vi "onenote_dialogue.vi"(8 "error in (no error)":errorcluster, 11 "Image Path":path=path "C:/Users/monke/Desktop/Work/VIs to modify/ONENOTE/Sandbox/TEST.BMP") -> (0 "error out":errorcluster, 2 "Description Out":string, 3 "Image Path Out":path)   [LabVIEW 2016]
uses:
  <vilib>/Utility/miscctls.llb/LVBoundsTypeDef.ctl
panel:
  in  "Options_Cluster":T1
  in  "Options":bool
  out "new picture":picture
  in  "Description":string="Write your description here. \nTo make text bold in OneNote, surround with <b><b/> tags.\nTo make text bold in OneNote, surround with <i><i/> tags."
  in  "Finish":bool
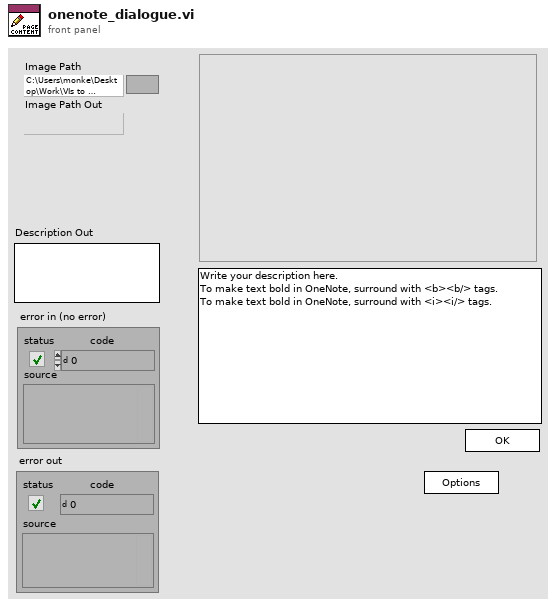
[diagram p1: front panel]
types:
  T1 = cluster{"Strikethrough":bool, "SubScript":bool, "Italics":bool, "Bold":bool, "SuperScript":bool}
  T2 = typedef "LVBoundsTypeDef.ctl" = cluster{"Width":u32, "Height":u32}
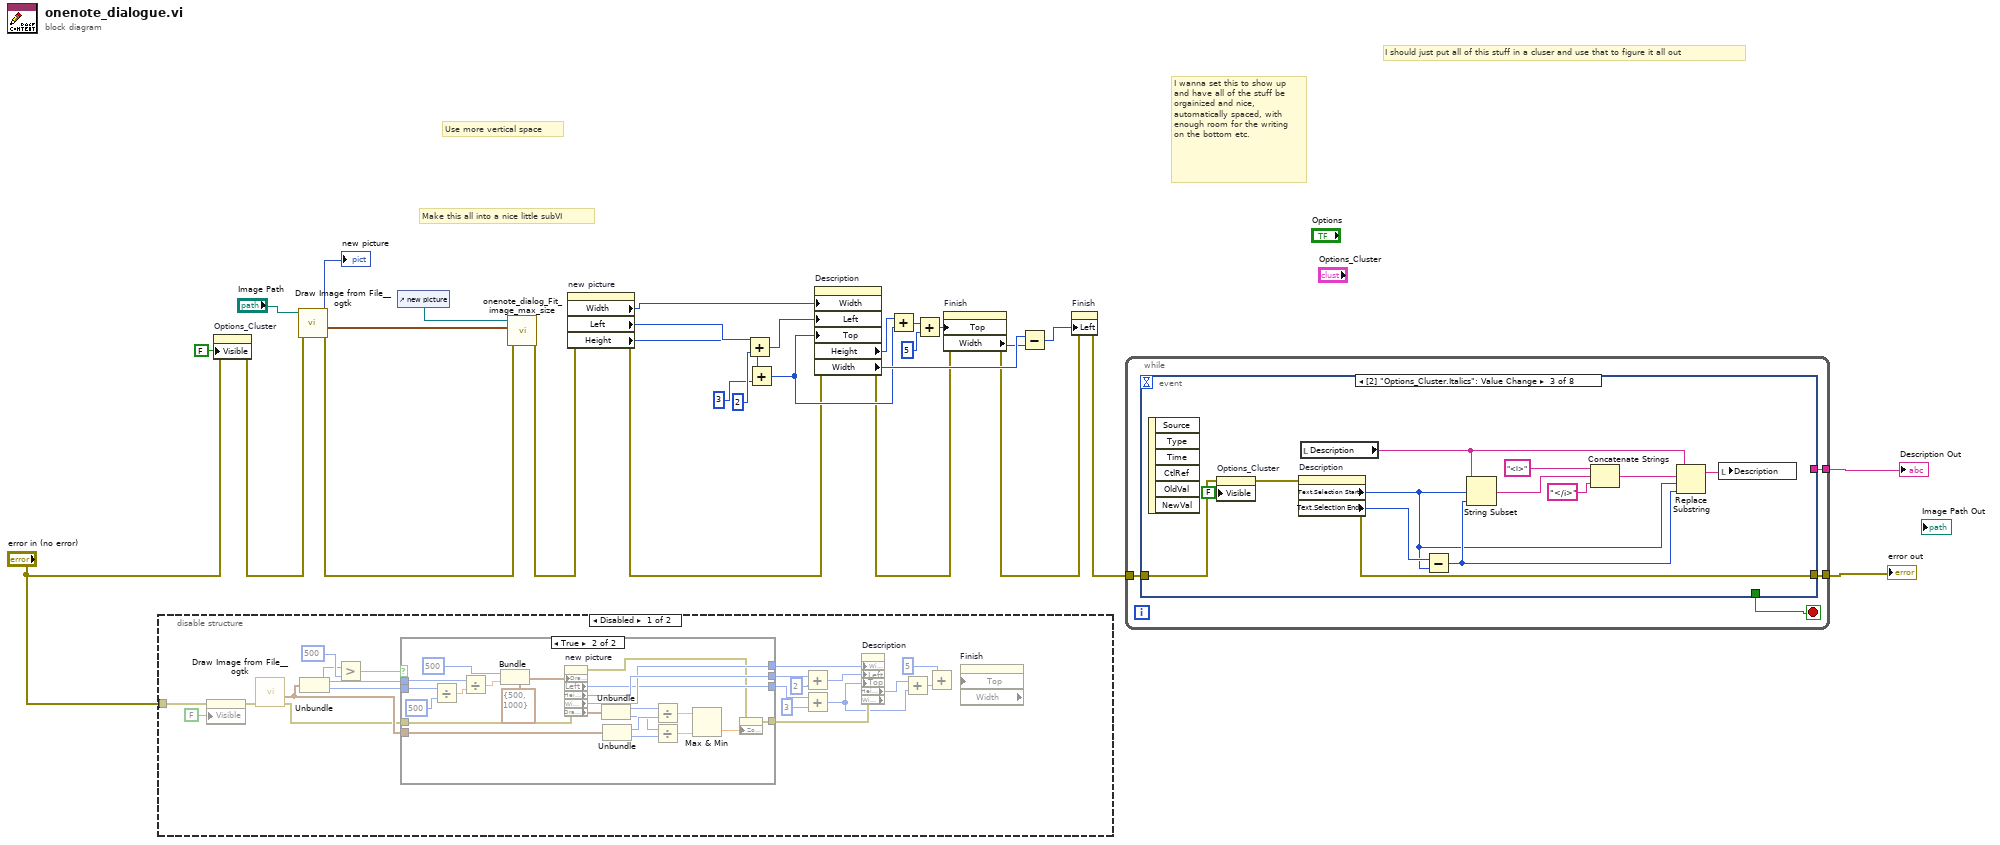
[diagram p0: block diagram]
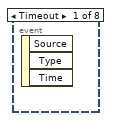
[diagram p4: hidden frame]
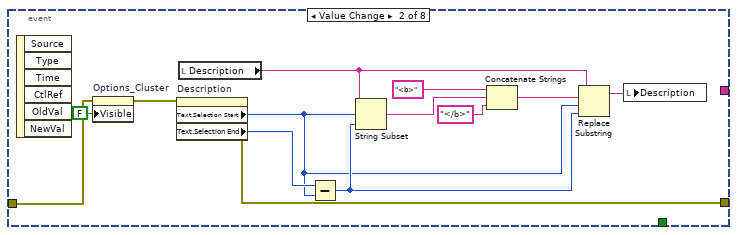
[diagram p5: hidden frame]
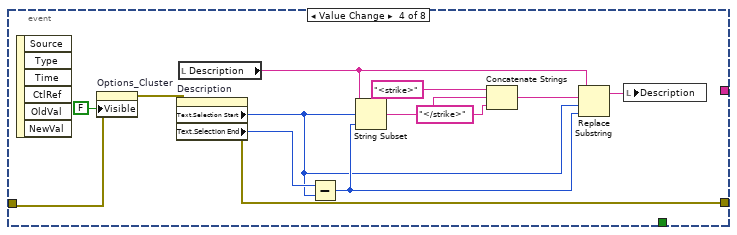
[diagram p6: hidden frame]
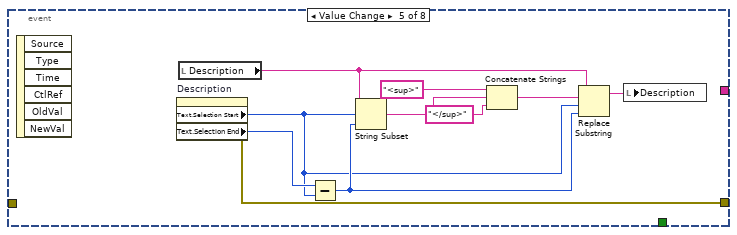
[diagram p7: hidden frame]
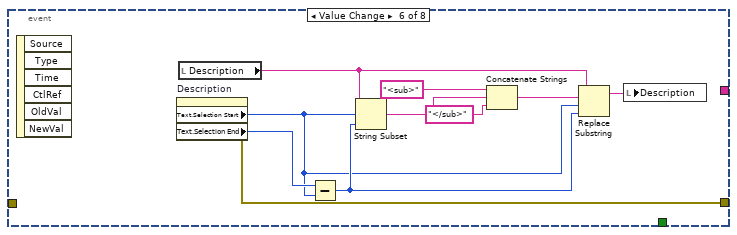
[diagram p8: hidden frame]
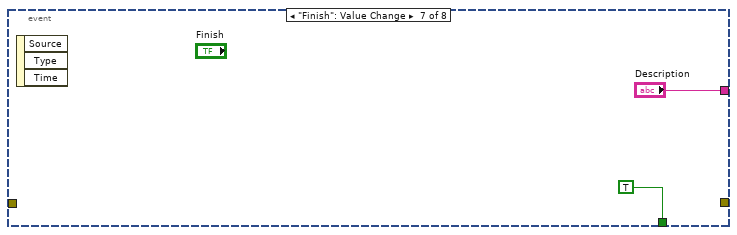
[diagram p9: hidden frame]
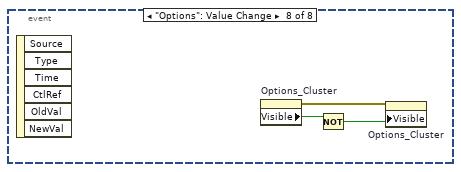
[diagram p10: hidden frame]
diagram:
  # "Make this all into a nice little subVI"
  # "Use more vertical space"
  # "I should just put all of this stuff in a cluser and use that to figure it all out"
  # "I wanna set this to show up and have all of the stuff be orgainized and nice, automatically spaced, with enough room for the writing on the bottom etc."
  n1 = disable-structure shown="Disabled" {
    disable-tunnel: "error in (no error)" -> [w43 _]
    frame Disabled {
      n2 = property on="Options_Cluster" class="Clust"(error in=w43, "Visible"=FALSE) -> (error out=w49:errorcluster)  [unwired: 1 in, 1 out]
      n3 = call <userlib>:"Draw Image from File__ogtk.vi"("error in (no error)"=w49) -> ("error out"=w34:errorcluster, "image size (pixels)"=w44:cluster{"x":i16, "y":i16})  [unwired: 7 in, 2 out]
      n4 = Unbundle(w44) -> ("x"=w46:i16, "y"=w45:i16)
      n5 = Greater?(x=w46, y=i16 500) -> (0:w47:bool)
      n6 = case shown="True" w47 {
        tunnel: w46 -> [_ w71]
        tunnel: w45 -> [_ w70]
        tunnel: w44 -> [_ w63]
        tunnel: [_ w54] -> w37
        tunnel: [_ w55] -> w41
        tunnel: [_ w53] -> w40
        tunnel: [_ w52] -> w35
        tunnel: w34 -> [_ w50]
        frame False {
        }
        frame True {
          n7 = Divide(x=w70, y=i16 500) -> (x/y=w72:dbl)
          n8 = Divide(x=w71, y=w72) -> (x/y=w66:dbl)
          n9 = Bundle(cluster=T2 {"Width"=500, "Height"=1000} ("Draw Area Size"), "Width"=u32 500, "Height"=w66) -> (w65:T2)
          n10 = property on="new picture" class="Pict"(error in=w50, "Draw Area Size"=w65) -> (error out=w51:errorcluster, "Left"=w53:i32, "Height"=w55:u32, "Width"=w54:u32, "Draw Area Size"=w64:T2)  [unwired: 1 in, 1 out]
          n11 = Unbundle(w64) -> ("Width"=w61:u32, "Height"=w60:u32)
          n12 = Unbundle(w63) -> ("x"=w62:i16, "y"=w59:i16)
          n13 = Divide(x=w61, y=w62) -> (x/y=w58:dbl)
          n14 = Divide(x=w60, y=w59) -> (x/y=w57:dbl)
          n15 = Max & Min(x=w58, y=w57) -> (min(x,y)=w56:dbl)  [unwired: 1 out]
          n16 = property on="new picture" class="Pict"(error in=w51, "ZoomFactor"=w56) -> (error out=w52:errorcluster)  [unwired: 1 in, 1 out]
        }
      }
      n17 = Add(x=w41, y=u32 2) -> (x+y=w36:u32)
      n18 = Add(x=w40, y=u32 3) -> (x+y=w32:u32)
      n19 = property on="Description" class="Str" props=["Width", "Left", "Top", "Height", "Width"](error in=w35, "Width"=w37, "Left"=w36, "Top"=w32) -> ("Height"=w33:u32)  [unwired: 1 in, 3 out]
      n20 = Add(x=w33, y=w32) -> (x+y=w31:u32)
      n21 = Add(x=u32 5, y=w31) -> ()  [unwired: 1 out]
      n22 = property on="Finish" class="Bool" props=["Top", "Width"]() -> ()  [unwired: 3 in, 3 out]
    }
    frame Enabled {
    }
  }
  n23 = property on="Options_Cluster" class="Clust"(error in="error in (no error)", "Visible"=FALSE) -> (error out=w11:errorcluster)  [unwired: 1 in, 1 out]
  n24 = call <userlib>:"Draw Image from File__ogtk.vi"("error in (no error)"=w11, "path to image file"="Image Path") -> ("error out"=w8:errorcluster, "image size (pixels)"=w7:cluster{"x":i16, "y":i16}, "new picture"=→"new picture":picture)  [unwired: 6 in, 1 out]
  n25 = control-ref of="new picture"() -> (w6:refnum<vi>)
  n26 = call "onenote_dialog_Fit_image_max_size.vi"("error in (no error)"=w8, "image size (pixels)"=w7, "Picture Refnum"=w6) -> ("error out"=w4:errorcluster)  [unwired: 8 in]
  n27 = property on="new picture" class="Pict"(error in=w4) -> (error out=w3:errorcluster, "Width"=w5:u32, "Left"=w2:i32, "Height"=w1:u32)  [unwired: 1 in, 1 out]
  n28 = Add(x=w2, y=2) -> (x+y=w10:i32)
  n29 = Add(x=w1, y=u32 3) -> (x+y=w17:u32)
  n30 = property on="Description" class="Str"(error in=w3, "Width"=w5, "Left"=w10, "Top"=w17) -> (error out=w14:errorcluster, "Height"=w18:u32, "Width"=w22:u32)  [unwired: 1 in, 1 out]
  n31 = Add(x=w18, y=w17) -> (x+y=w23:u32)
  n32 = Add(x=w23, y=u32 5) -> (x+y=w24:u32)
  n33 = property on="Finish" class="Bool"(error in=w14, "Top"=w24) -> (error out=w13:errorcluster, "Width"=w21:u32)  [unwired: 1 in, 1 out]
  n34 = Subtract(x=w22, y=w21) -> (x-y=w16:u32)
  n35 = property on="Finish" class="Bool"(error in=w13, "Left"=w16) -> (error out=w12:errorcluster)  [unwired: 1 in, 1 out]
  n36 = while {
    tunnel: [w75] -> w20
    tunnel: [w74] -> w19
    tunnel: w12 -> [w73]
    stop <- w76 stop-if-true
    n37 = event shown="[2] \"Options_Cluster.Italics\": Value Change" {
      selector: _ -> [_ _ _ _ _ _ _ _]
      dyn-events: _ -> [_ _ _ _ _ _ _ _]
      timeout: _ -> [_ _ _ _ _ _ _ _]
      tunnel: [_ _ _ _ _ _ TRUE _] -> w76
      tunnel: [_ _ _ _ _ _ "Description" _] -> w75
      tunnel: [_ w83 w96 w109 w119 w129 _ _] -> w74
      tunnel: w73 -> [_ w78 w91 w103 _ _ _ _]
      event Timeout {
        n38 = event-data() -> ()  [unwired: 1 in, 3 out]
      }
      event "Options_Cluster.Bold": Value Change {
        n39 = event-data() -> ()  [unwired: 1 in, 6 out]
        n40 = property on="Options_Cluster" class="Clust"(error in=w78, "Visible"=FALSE) -> (error out=w79:errorcluster)  [unwired: 1 in, 1 out]
        n41 = property on="Description" class="Str"(error in=w79) -> (error out=w83:errorcluster, "Text.Selection Start"=w80:u32, "Text.Selection End"=w89:u32)  [unwired: 1 in, 1 out]
        n42 = local read "Description"() -> (w81:string)
        n43 = Subtract(x=w89, y=w80) -> (x-y=w87:u32)
        n44 = String Subset(string=w81, offset (0)=w80, length (rest)=w87) -> (substring=w85:string)
        n45 = Concatenate Strings("<b>" ("string"), w85, "</b>" ("string")) -> (w88:string)
        n46 = Replace Substring(2:w87, 3:w80, 4:w88, 5:w81) -> (1:w84:string)  [unwired: 1 out]
        n47 = local write "Description"(w84) -> ()
      }
      event "Options_Cluster.Italics": Value Change {
        n48 = event-data() -> ()  [unwired: 1 in, 6 out]
        n49 = property on="Options_Cluster" class="Clust"(error in=w91, "Visible"=FALSE) -> (error out=w92:errorcluster)  [unwired: 1 in, 1 out]
        n50 = property on="Description" class="Str"(error in=w92) -> (error out=w96:errorcluster, "Text.Selection Start"=w93:u32, "Text.Selection End"=w102:u32)  [unwired: 1 in, 1 out]
        n51 = local read "Description"() -> (w94:string)
        n52 = Subtract(x=w102, y=w93) -> (x-y=w100:u32)
        n53 = String Subset(string=w94, offset (0)=w93, length (rest)=w100) -> (substring=w98:string)
        n54 = Concatenate Strings("<i>" ("string"), w98, "</i>" ("string")) -> (w101:string)
        n55 = Replace Substring(2:w100, 3:w93, 4:w101, 5:w94) -> (1:w97:string)  [unwired: 1 out]
        n56 = local write "Description"(w97) -> ()
      }
      event "Options_Cluster.Strikethrough": Value Change {
        n57 = event-data() -> ()  [unwired: 1 in, 6 out]
        n58 = property on="Options_Cluster" class="Clust"(error in=w103, "Visible"=FALSE) -> (error out=w105:errorcluster)  [unwired: 1 in, 1 out]
        n59 = property on="Description" class="Str"(error in=w105) -> (error out=w109:errorcluster, "Text.Selection Start"=w106:u32, "Text.Selection End"=w115:u32)  [unwired: 1 in, 1 out]
        n60 = local read "Description"() -> (w107:string)
        n61 = Subtract(x=w115, y=w106) -> (x-y=w113:u32)
        n62 = String Subset(string=w107, offset (0)=w106, length (rest)=w113) -> (substring=w111:string)
        n63 = Concatenate Strings("<strike>" ("string"), w111, "</strike>" ("string")) -> (w114:string)
        n64 = Replace Substring(2:w113, 3:w106, 4:w114, 5:w107) -> (1:w110:string)  [unwired: 1 out]
        n65 = local write "Description"(w110) -> ()
      }
      event "Options_Cluster.SuperScript": Value Change {
        n66 = event-data() -> ()  [unwired: 1 in, 6 out]
        n67 = property on="Description" class="Str"() -> (error out=w119:errorcluster, "Text.Selection Start"=w116:u32, "Text.Selection End"=w125:u32)  [unwired: 2 in, 1 out]
        n68 = local read "Description"() -> (w117:string)
        n69 = Subtract(x=w125, y=w116) -> (x-y=w123:u32)
        n70 = String Subset(string=w117, offset (0)=w116, length (rest)=w123) -> (substring=w121:string)
        n71 = Concatenate Strings("<sup>" ("string"), w121, "</sup>" ("string")) -> (w124:string)
        n72 = Replace Substring(2:w123, 3:w116, 4:w124, 5:w117) -> (1:w120:string)  [unwired: 1 out]
        n73 = local write "Description"(w120) -> ()
      }
      event "Options_Cluster.SubScript": Value Change {
        n74 = event-data() -> ()  [unwired: 1 in, 6 out]
        n75 = property on="Description" class="Str"() -> (error out=w129:errorcluster, "Text.Selection Start"=w126:u32, "Text.Selection End"=w135:u32)  [unwired: 2 in, 1 out]
        n76 = local read "Description"() -> (w127:string)
        n77 = Subtract(x=w135, y=w126) -> (x-y=w133:u32)
        n78 = String Subset(string=w127, offset (0)=w126, length (rest)=w133) -> (substring=w131:string)
        n79 = Concatenate Strings("<sub>" ("string"), w131, "</sub>" ("string")) -> (w134:string)
        n80 = Replace Substring(2:w133, 3:w126, 4:w134, 5:w127) -> (1:w130:string)  [unwired: 1 out]
        n81 = local write "Description"(w130) -> ()
      }
      event "Finish": Value Change {
        n82 = event-data() -> ()  [unwired: 1 in, 3 out]
      }
      event "Options": Value Change {
        n83 = event-data() -> ()  [unwired: 1 in, 6 out]
        n84 = property on="Options_Cluster" class="Clust"() -> (error out=w138:errorcluster, "Visible"=w140:bool)  [unwired: 2 in, 1 out]
        n85 = Not(x=w140) -> (.not. x?=w139:bool)
        n86 = property on="Options_Cluster" class="Clust"(error in=w138, "Visible"=w139) -> ()  [unwired: 1 in, 2 out]
      }
    }
  }
  "error out" <- w19
  "Description Out" <- w20
